vi "Test_Run and Refresh.vi"() -> ()   [LabVIEW 2019]
uses:
  AutoMenuCreator.lvlib
panel:
  out "Created mnu file paths":path[](array[path])
  out "error out":errorcluster
  in  "Target Folder":path=path "C:/Program Files (x86)/National Instruments/LabVIEW 2019/user.lib/_Tools/Tools.Application"
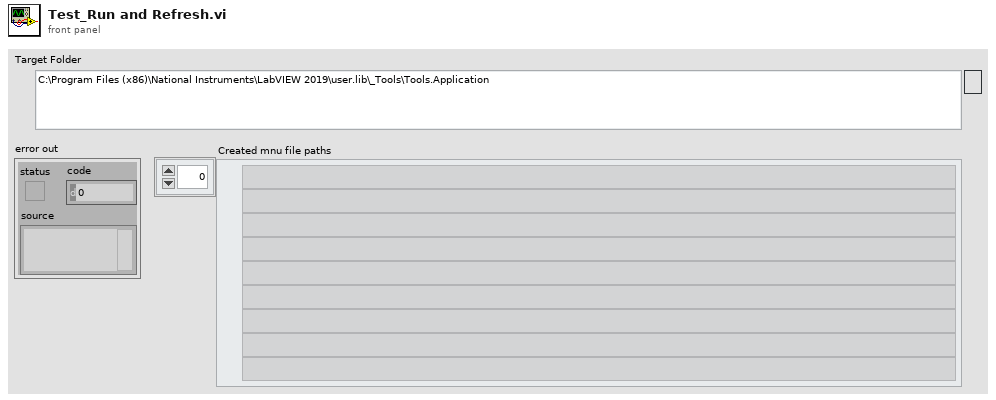
[diagram p1: front panel]
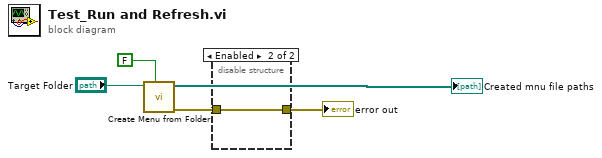
[diagram p0: block diagram]
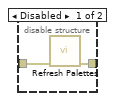
[diagram p2: hidden frame]
diagram:
  n1 = call "Create Menu from Folder.vi"("Allow Initialization of AutoMenu on Target(T)"=FALSE, "Target Folder"="Target Folder") -> ("error out"=w3:errorcluster, "Created mnu file paths"=→"Created mnu file paths":path[])  [unwired: 8 in]
  n2 = disable-structure shown="Enabled" {
    disable-tunnel: w3 -> [w7 w8]
    disable-tunnel: [w6 w8] -> w2
    frame Disabled {
      n3 = call "Refresh Palettes.vi"("error in (no error)"=w7) -> ("error out"=w6:errorcluster)  [unwired: 10 in]
    }
    frame Enabled {
    }
  }
  "error out" <- w2
